vi "工具选板.vi"() -> ()   [LabVIEW 2013]
panel:
  in  "?":bool
  out "?":bool
  out "?":bool
  out "?":bool
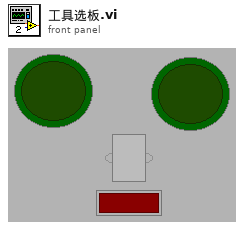
[diagram p1: front panel]
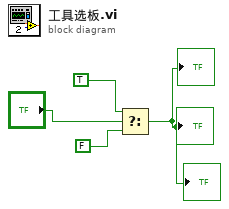
[diagram p0: block diagram]
diagram:
  n1 = Select(t=TRUE, s="?", f=FALSE) -> (s? t:f=→"?" →"?" →"?":bool)
